vi "Initialize.vi"(8 "error in (no error)":errorcluster, 11 "HSMS Class":refnum<class "HSMS Class.lvclass">) -> (0 "error out":errorcluster, 3 "Scenarios Class out":refnum<class "Scenarios Class.lvclass">)   [LabVIEW 2020, in "SECS Scenarios.lvlib" / "Scenarios Class.lvclass"]
uses:
  Scenarios Class.lvclass
  SECS Communication/HSMS Class/HSMS Class.lvclass
  Scenarios Class.lvclass/Scenarios Class.ctl
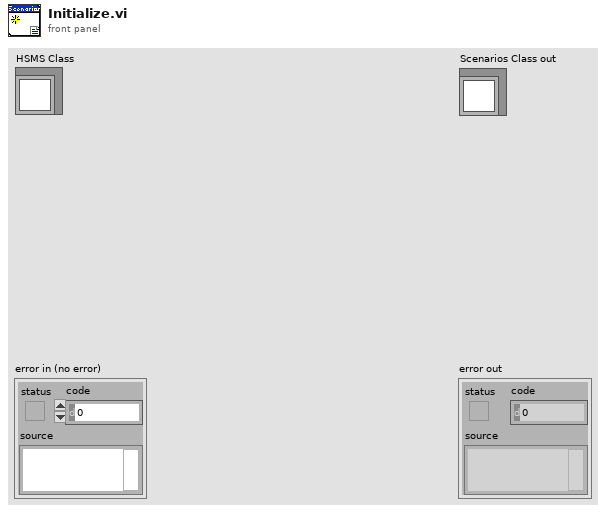
[diagram p1: front panel]
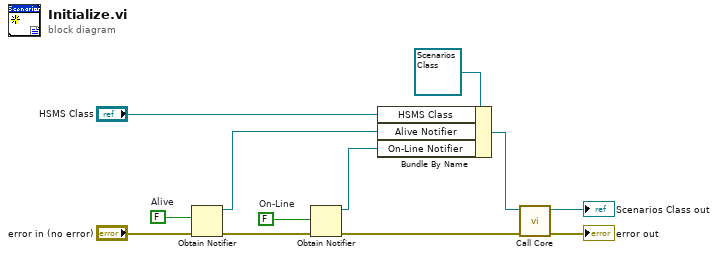
[diagram p0: block diagram]
diagram:
  w4 = FALSE  # On-Line
  w9 = FALSE  # Alive
  n1 = Obtain Notifier(notification data type=w9, error in (no error)="error in (no error)") -> (notifier out=w8:refnum<notifier>, error out=w3:errorcluster)  [unwired: 2 in, 1 out]
  n2 = Obtain Notifier(notification data type=w4, error in (no error)=w3) -> (notifier out=w2:refnum<notifier>, error out=w1:errorcluster)  [unwired: 2 in, 1 out]
  n3 = Bundle By Name(cluster=refnum<class "Scenarios Class.lvclass"> refnum ("Scenarios Class in"), "HSMS Class"="HSMS Class", "Alive Notifier"=w8, "On-Line Notifier"=w2) -> (w7:refnum<class "Scenarios Class.lvclass">)
  n4 = call "Call Core.vi"("error in (no error)"=w1, "Scenarios Class in"=w7) -> ("error out"=→"error out":errorcluster, "Scenarios Class out"=→"Scenarios Class out":refnum<class "Scenarios Class.lvclass">)  [unwired: 8 in]
